vi "Create-action.vi"(8 "error in (no error)":errorcluster, 10 "Action":string) -> (0 "error out":errorcluster, 3 "Action out":refnum<class "Action.lvclass">)   [LabVIEW 2013, in "Messages.lvlib" / "Action.lvclass"]
uses:
  Action.lvclass
  Base-messages.ctl
  Action.lvclass/Action.ctl
  Messages.lvlib
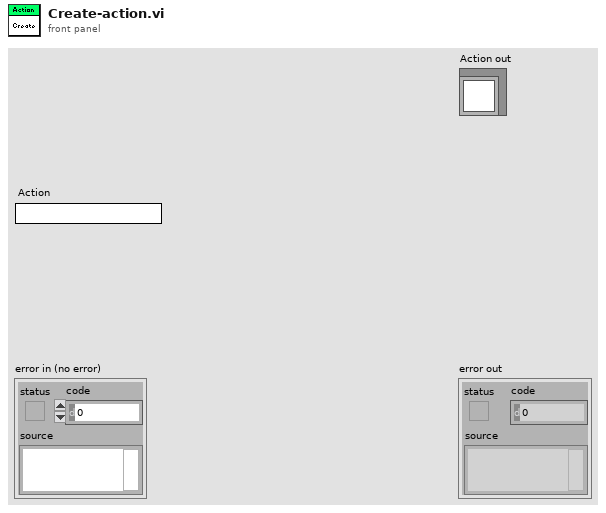
[diagram p1: front panel]
types:
  T1 = typedef "Messages.lvlib/Base-messages.ctl" = enum16{"Heartbeat", "Error", "Start client", "Stop client", "Get clients", "Query status", "Send status", "Action"}
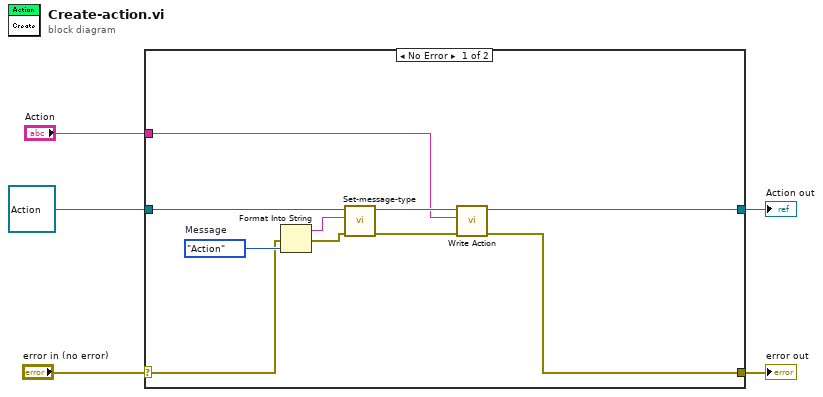
[diagram p0: block diagram]
diagram:
  n1 = case shown="No Error" "error in (no error)" {
    selector: "error in (no error)" -> [w11 w17]
    tunnel: [w6 w17] -> w4
    tunnel: [w7 w16] -> w3
    tunnel: refnum<class "Action.lvclass"> refnum ("Message in") -> [w15 w16]
    tunnel: "Action" -> [w8 _]
    frame No Error {
      w14 = Base-messages."Action"  # Message
      n2 = Format Into String(error in=w11, w14) -> (resulting string=w13:string, error out=w12:errorcluster)  [unwired: 2 in]
      n3 = call-dynamic "Set-message-type.vi"("error in (no error)"=w12, "Message type"=w13, "Message in"=w15) -> ("error out"=w9:errorcluster, "Message out"=w10:refnum<class "Action.lvclass">)  [unwired: 7 in]
      n4 = call "Write Action.vi"("error in (no error)"=w9, "Action"=w8, "Action in"=w10) -> ("error out"=w6:errorcluster, "Action out"=w7:refnum<class "Action.lvclass">)  [unwired: 7 in]
    }
    frame Error {
    }
  }
  "error out" <- w4
  "Action out" <- w3
